vi "sensor input.vi"() -> ()   [LabVIEW 2019]
uses:
  <vilib>/addons/control/pid/pid.llb/PID (DBL).vi
  <vilib>/Analysis/NI_AALBase.lvlib
  <vilib>/addons/control/pid/NI_PID_pid.lvlib
  <vilib>/ptbypt/NI_PtbyPt.lvlib
panel:
  out "Waveform Chart 2":dbl(graph)
  out "Waveform Chart":dbl[][](graph)
  in  "PID gains":T1={"proportional gain (Kc)"=0.001, "integral time (Ti, min)"=30.0, "derivative time (Td, min)"=0.0} {"derivative time (Td, min)" format="%.3f"; "integral time (Ti, min)" format="%.3f"; "proportional gain (Kc)" format="%.3f"}
  out "PWM Output":bool
  in  "Slide":dbl(slide) scale=0.0..10.0
  out "Waveform Graph 2":dbl[](graph)
  in  "stop (F)":bool
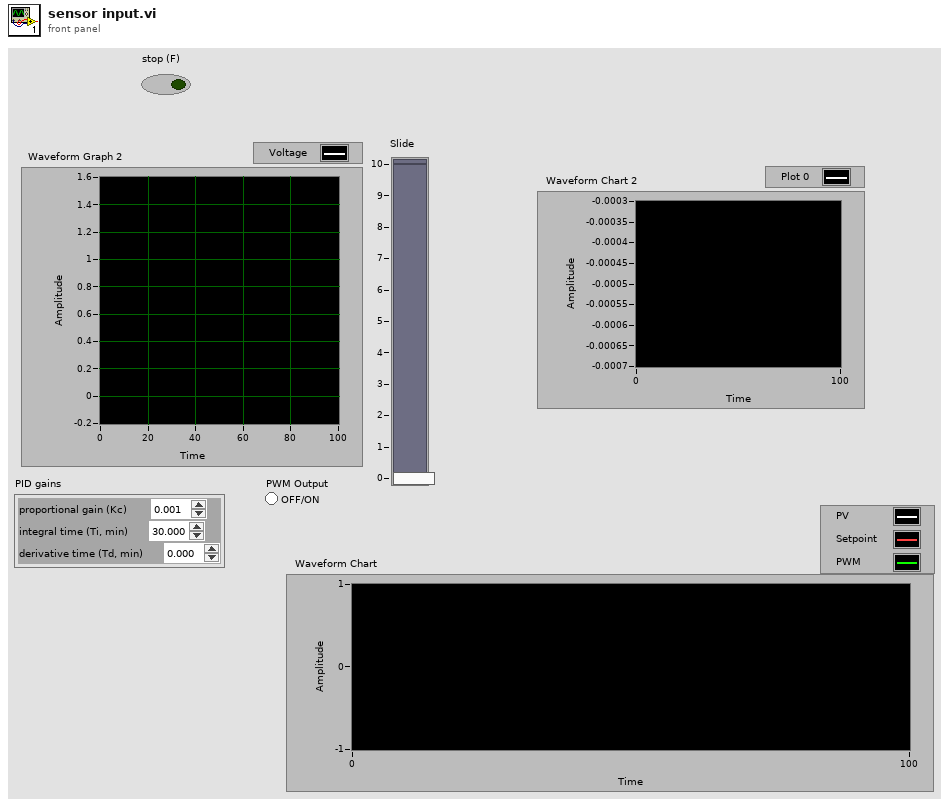
[diagram p1: front panel]
types:
  T1 = cluster{"proportional gain (Kc)":dbl, "integral time (Ti, min)":dbl, "derivative time (Td, min)":dbl}
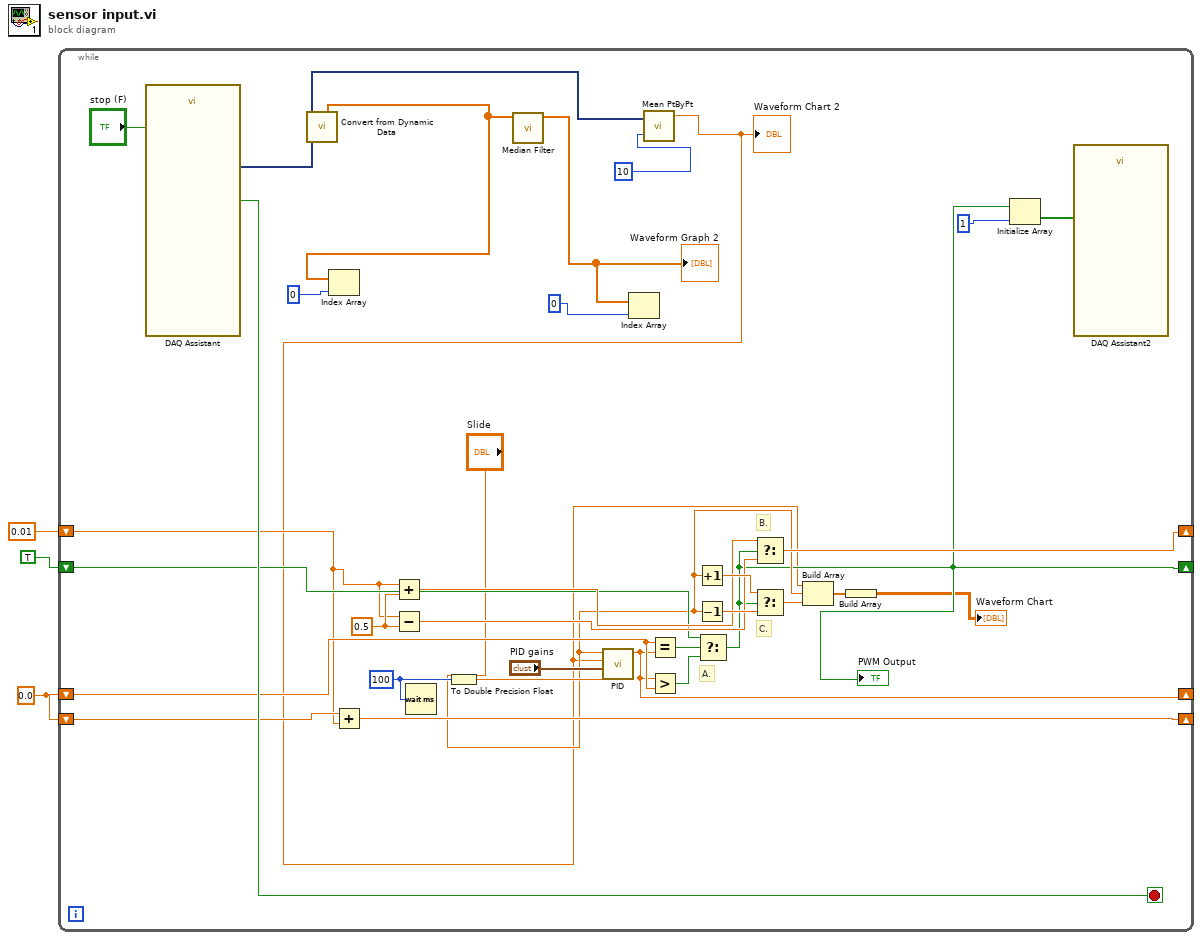
[diagram p0: block diagram]
diagram:
  w3 = 0.0 ("output")
  n1 = while {
    shift-right: [w18] -> _
    shift-left: w3 -> [w19]
    shift-right: [w16] -> _
    shift-left: w3 -> [w17]
    shift-right: [w11] -> _
    shift-left: TRUE -> [w15]
    shift-right: [w14] -> _
    shift-left: 0.01 -> [w13]
    stop <- w33 stop-if-true
    w22 = 0.5 ("x")
    w30 = u32 100 ("milliseconds to wait")
    # "B."
    # "C."
    # "A."
    n2 = call "DAQ Assistant"("stop (F)"="stop (F)") -> ("data"=w6:dynamicdata, "stopped"=w33:bool)  [unwired: 15 in, 2 out]
    n3 = call "Convert from Dynamic Data"("Dynamic Data Type"=w6) -> ("Array"=w9:dbl[])  [unwired: 3 in]
    n4 = Index Array(array=w9, index=0) -> ()  [unwired: 1 out]
    n5 = Add(x=w19, y=w13) -> (x+y=w18:dbl)
    n6 = Add(x=w13, y=w22) -> (x+y=w23:dbl)
    n7 = Subtract(x=w13, y=w22) -> (x-y=w21:dbl)
    n8 = Wait (ms)(milliseconds to wait=w30) -> ()  [unwired: 1 out]
    n9 = To Double Precision Float(number=w30) -> (double precision float=w20:dbl)
    n10 = call <vilib>:"Median Filter.vi"("X"=w9) -> ("Filtered X"=w8:dbl[])  [unwired: 9 in, 1 out]
    "Waveform Graph 2" <- w8
    n11 = Index Array(array=w8, index=0) -> ()  [unwired: 1 out]
    n12 = call <vilib>:"Mean PtByPt.vi"("x"=w6, "sample length"=10 ("index")) -> ("mean"=w4:dbl)  [unwired: 2 in, 1 out]
    "Waveform Chart 2" <- w4
    n13 = call-poly <vilib>:"PID.vi"("dt (s)"=w20, "PID gains"="PID gains", "process variable"=w4, "setpoint"="Slide") -> ("output"=w16:dbl)  [unwired: 6 in, 1 out]
    n14 = Equal?(x=w17, y=w16) -> (x = y?=w29:bool)
    n15 = Greater?(x=w16, y=w17) -> (0:w28:bool)
    n16 = Increment(x="Slide") -> (x+1=w27:dbl)
    n17 = Decrement(x="Slide") -> (x-1=w26:dbl)
    n18 = Select(t=w15, s=w29, f=w28) -> (s? t:f=w11:bool)
    "PWM Output" <- w11
    n19 = Select(t=w23, s=w11, f=w21) -> (s? t:f=w14:dbl)
    n20 = Select(t=w27, s=w11, f=w26) -> (s? t:f=w25:dbl)
    n21 = Build Array(w4, "Slide", w25) -> (w24:dbl[])
    n22 = Build Array(w24) -> (→"Waveform Chart":dbl[][])
    n23 = Initialize Array(w11, 1 ("dimension size")) -> (w32:bool[])
    n24 = call "DAQ Assistant2"("data"=w32) -> ()  [unwired: 17 in, 2 out]
  }
